vi "Read connection_timeout .vi"(8 "error in (no error)":errorcluster, 11 "TCPSettings in":refnum<class "TCPSettings.lvclass">) -> (0 "error out":errorcluster, 2 "connection_timeout":i32=10, 3 "TCPSettings out":refnum<class "TCPSettings.lvclass">)   [LabVIEW 2016, in "TCPSettings.lvclass"]
uses:
  TCPSettings.lvclass
  TCPSettings.lvclass/TCPSettings.ctl
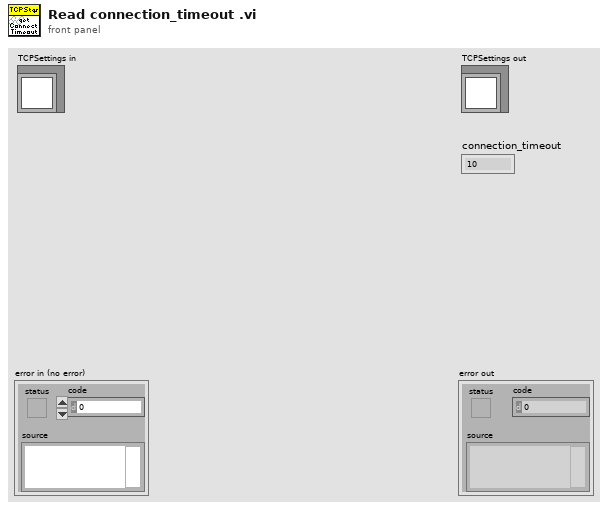
[diagram p1: front panel]
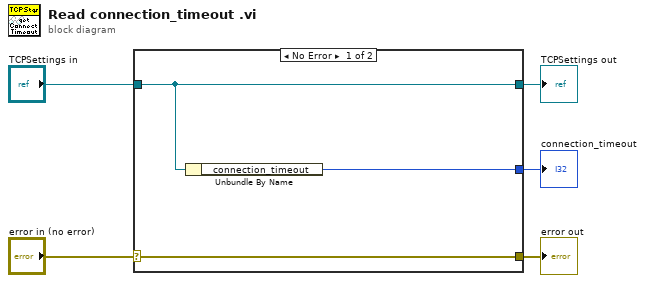
[diagram p0: block diagram]
diagram:
  n1 = case shown="No Error" "error in (no error)" {
    selector: "error in (no error)" -> [w8 w9]
    tunnel: [w8 w9] -> w4
    tunnel: [w7 w10] -> w2
    tunnel: "TCPSettings in" -> [w7 w10]
    tunnel: [w6 _] -> w1
    frame No Error {
      n2 = Unbundle By Name(w7) -> ("connection_timeout"=w6:i32)
    }
    frame Error {
    }
  }
  "error out" <- w4
  "TCPSettings out" <- w2
  "connection_timeout" <- w1
